vi "Main v1.6.vi"() -> ()   [LabVIEW 2017]
doc: "v0.85:\n- Counts for rejects and total\n\nv0.5:\n\n- Added Reject to Manual Mode\n- Send reject pallet cluster during manual mode\n- Run continuous manual happens only when no error has occured"
uses:
  Controls/Main Tabs v0.1.ctl
  Controls/Auto.ctl
  RT/Controls/Auto Delays.ctl
  RT/Controls/Auto Times.ctl
  support/Controls/General Para.ctl
  support/Message Queue/Message Cluster.ctl
  Controls/UI Data.ctl
  support/Controls/Auto Stats.ctl
  Controls/Logging FGV.ctl
  support/Message Queue/Enqueue Message (Single).vi
  GV/Maintenance GV.vi
  <vilib>/Utility/error.llb/Error Cluster From Error Code.vi
  <vilib>/ErrorRing/Error Ring.xnode
  support/Message Queue/Message Queue.lvlib
  support/User Event - Stop/User Event - Stop.lvlib
panel:
  in  "dup Message Queue":refnum<queue>
  out "path":path
  in  "General Para 2":T1={"Max. Cons."=5.0, "Offset 1"=0.0, "Offset 2"=0.0, "Offset 3"=0.0, "Offset 4"=-0.6, "OutputPause"=500.0, "RejectPause"=500.0} caption="General Para" {"Offset 4" format="%.2f"; "Offset 3" format="%.2f"; "Offset 2" format="%.2f"; "Offset 1" format="%.2f"}
  in  "Auto Para 2":T2={"Agitator Delays"=[250, 600], "TF Delays"=[400, 800, 2, 8000], "Insertion Delays"=[100, 400], "Cutting Delays"=[200, 300, 50], "PF Delays"=[300, 8000], "Measur. Delays"=[200.0, 188.9, 1.0], "Reject Delays"=[500], "BF Delays"=[1000, 1000]}
  out "Shutdown?":bool
  out "Boolean 8":bool
  out "Boolean 7":bool
  out "Boolean 6":bool
  out "Boolean 5":bool
  out "Boolean 4":bool
  out "Boolean 3":bool
  out "Boolean 2":bool
  out "Boolean":bool
  in  "Reject Pallets":T3
  out "Date-Time":string caption="Dip-Tube Assembly Automation (HMI) v1.6"
  out "Main Tab":T4
  in  "All IOs":bool
  in  "Autocycle":T5
  in  "Manual":bool
  in  "Parameters":bool
  in  "Maintenance":bool
  in  "General Para":T1={"Max. Cons."=5.0, "Offset 1"=0.0, "Offset 2"=0.0, "Offset 3"=0.0, "Offset 4"=0.0, "OutputPause"=0.0, "RejectPause"=0.0} {"Offset 4" format="%.2f"; "Offset 3" format="%.2f"; "Offset 2" format="%.2f"; "Offset 1" format="%.2f"}
  in  "BF Para":cluster{"Delay 1":u32, "Delay 2":u32}={"Delay 1"=1000, "Delay 2"=1000}
  in  "Reject Para":cluster{"Delay":u32}={"Delay"=400}
  in  "Meas. Para":T6={"Delay"=500.0, "Mean Length"=188.9, "Tolerance"=1.0}
  in  "PF Para":cluster{"Delay":u32, "Timeout":u32}={"Delay"=1000, "Timeout"=1000}
  in  "Tube Feeder Para":T7={"Delay"=400, "Delay 2"=250, "Max Attempts"=250, "Timeout"=8000}
  in  "Cutting Para":T8={"Delay"=400, "Delay 2"=250, "Delay 3"=250}
  in  "Agitator Para":cluster{"Delay":u32, "Timeout":u32}={"Delay"=400, "Timeout"=250}
  in  "Insertion Para":cluster{"Delay 1":u32, "Delay 2":u32}={"Delay 1"=1000, "Delay 2"=1000}
  in  "Save Para":bool
  in  "Home Para":bool
  out "OEE":dbl format="%#.1f"
  out "QUA":dbl=100.0 min=0.0 max=100.0 step=0.1
  in  "Ideal Time":dbl=2.0 min=0.0 max=100.0 step=0.1
  in  "AVL":dbl=100.0 min=0.0 max=100.0 step=0.1
  out "Rejects 2":u32 caption="Rejects"
  in  "Reset MCount":bool
  in  "Enable BF?":bool
  in  "Enable Agitate?":bool
  in  "Enable Reject?":bool
  in  "Toggle Motor":bool
  in  "Continuous?":bool
  in  "Enable Measure?":bool
  in  "Enable Index?":bool
  in  "Enable PF?":bool
  in  "Manual Para":T2={"Agitator Delays"=[400, 250], "TF Delays"=[700, 800, 2], "Insertion Delays"=[100, 500], "Cutting Delays"=[300, 300, 100], "PF Delays"=[250, 30000], "Measur. Delays"=[500.0, 188.9, 1.0], "Reject Delays"=[500], "BF Delays"=[1000, 1000]}
  in  "Enable Cutting?":bool
  in  "Enable Insertion?":bool
  in  "Run Manual":bool
  in  "Enable TF?":bool
  in  "Home Manual":bool
  out "Status 2":T10
  out "Measurements":T11 {"Height 1" format="%#.2f"; "Height 2" format="%#.2f"; "Height 3" format="%#.2f"; "Height 4" format="%#.2f"}
  out "Output Count":u32 caption="Output\nCount"
  out "PRF":dbl=100.0 min=0.0 max=100.0 step=0.1
  in  "ResetRejectCount":bool
  in  "ResetGoodCount":bool
  out "RejectPause":u32 caption="Reject Parts"
  out "GoodPause":u32 caption="Good Parts"
  in  "End Cycle":bool
  out "Statuses":string[][](table)
  in  "All IO":bool
  in  "Stats":bool
  in  "Home AC":bool
  out "Status":string
  out "Good":u32 format="%06.0f"
  out "Cycle Time":dbl format="%0.2f"
  out "Rejects":u32 format="%05.0f"
  in  "View Log":bool
  out "Total Count 2":u32 caption="Total Count"
  out "Avg. Time":dbl caption="Avg. Cycle Time (s)" format="%#.3f"
  out "Output Chart":cluster{"Good Parts":u32, "Reject Parts":u32}(graph)
  out "Reject Count":u32
  out "Good Count":u32
  out "Total Time":dbl caption="Effective Cycle Time (s)" format="%#.3f"
  out "Time Chart":T12(graph)
  out "OEE Chart":T13(graph)
  out "Timestamp":string caption="Date & Timestamp"
  out "Latest Measure.":T14 caption="Latest Measurements" {"Length 1 (mm)" format="%#.2f"}
  out "Auto Times":T9
  in  "Back Stats":bool
  out "OEE 2":T13 caption="Latest Measurements" {"AVL" format="%#.1f"; "PRF" format="%#.1f"; "QUA" format="%#.1f"; "OEE" format="%#.1f"}
  out "Measurement Chart":T15(graph)
  in  "Home IOs":bool
  in  "Back IO":bool
  out "IAS 4":dbl format="%#.3f"
  out "IAS 3":dbl format="%#.3f"
  out "IAS 2":dbl format="%#.3f"
  out "IAS 1":dbl format="%#.3f"
  out "DI 1":T16
  out "DI 2":T17
  out "DO 1":T18
  in  "Exit":bool
  in  "Shutdown":bool
  # "HARMONY VISION DIP-TUBE ASSEMBLY AUTOMATION"
  # "Auto-Pause after"
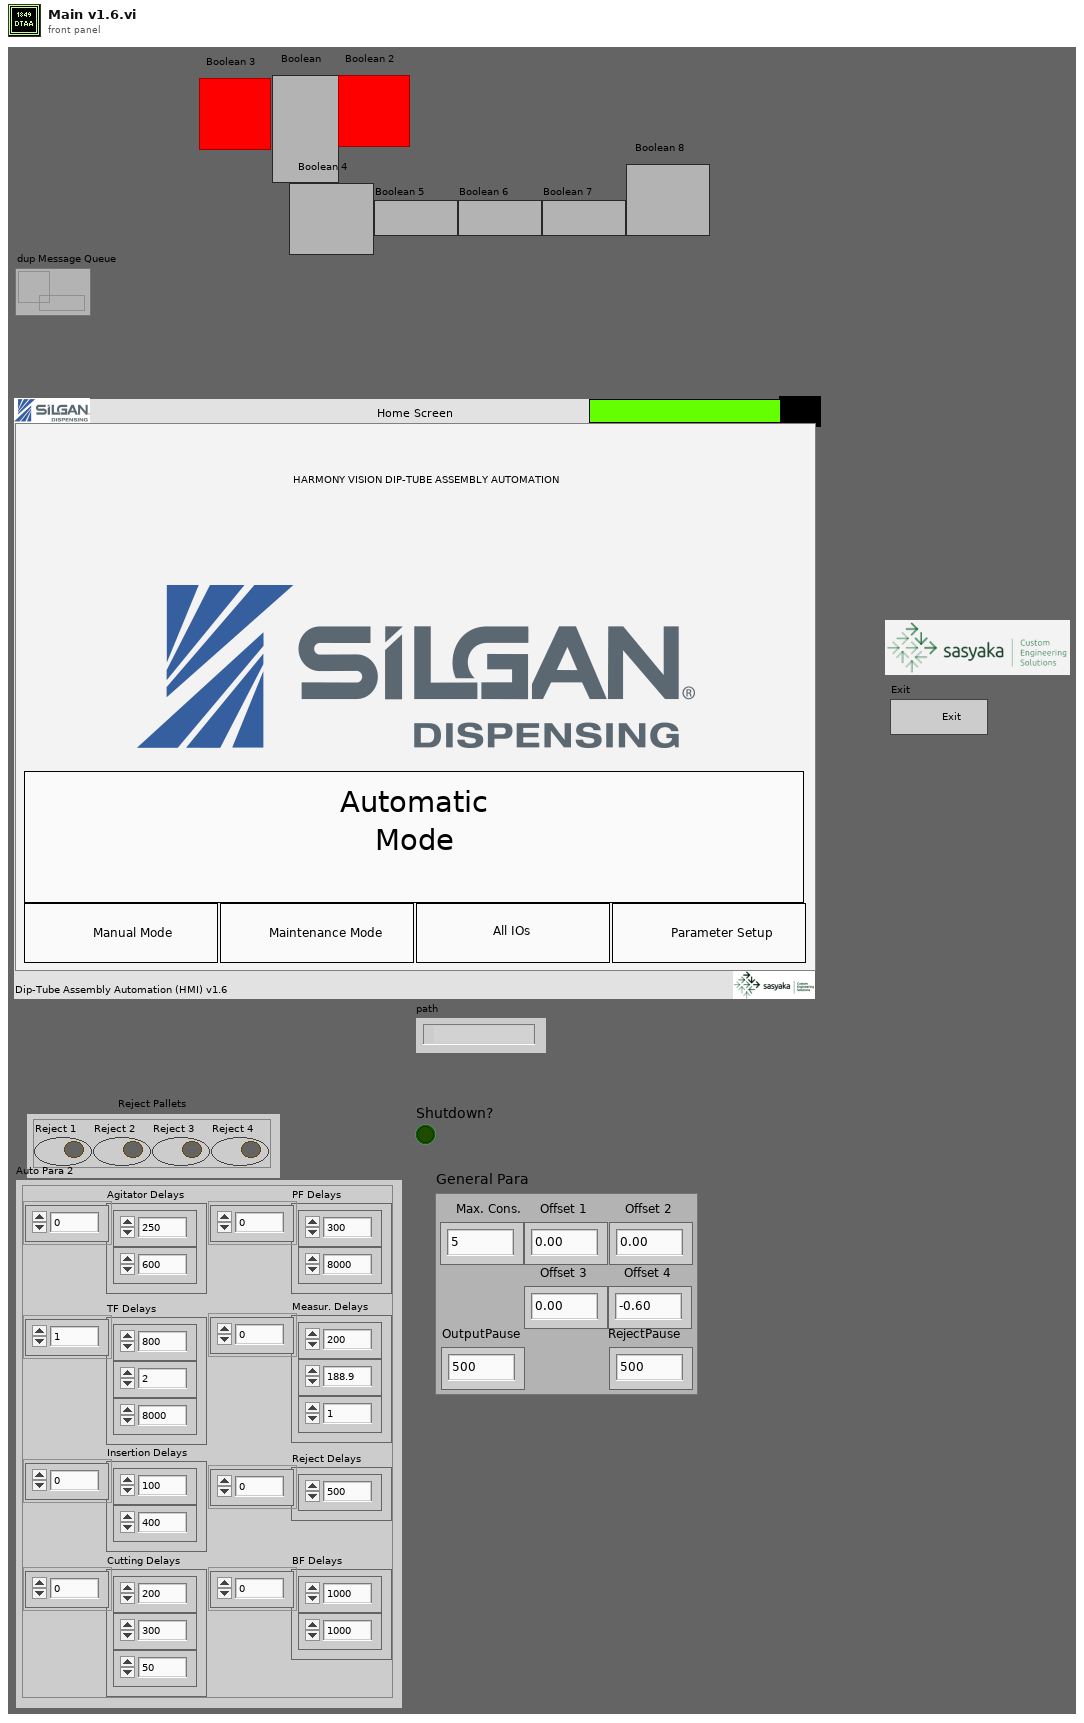
[diagram p1: front panel]
types:
  T1 = typedef "General Para.ctl" = cluster{"Max. Cons.":dbl, "Offset 1":dbl, "Offset 2":dbl, "Offset 3":dbl, "Offset 4":dbl, "OutputPause":dbl, "RejectPause":dbl}
  T2 = typedef "Auto Delays.ctl" = cluster{"Agitator Delays":u32[], "TF Delays":u32[], "Insertion Delays":u32[], "Cutting Delays":u32[], "PF Delays":u32[], "Measur. Delays":dbl[], "Reject Delays":u32[], "BF Delays":u32[]}
  T3 = cluster{"Reject 1":bool, "Reject 2":bool, "Reject 3":bool, "Reject 4":bool}
  T4 = typedef "Main Tabs v0.1.ctl" = enum32{"Home Screen", "Parameter Setup", "Manual Mode", "Autocycle", "Autocycle Statistics", "Autocycle IOs"}
  T5 = typedef "Auto.ctl" = bool
  T6 = cluster{"Delay":dbl, "Mean Length":dbl, "Tolerance":dbl}
  T7 = cluster{"Delay":u32, "Delay 2":u32, "Max Attempts":u32, "Timeout":u32}
  T8 = cluster{"Delay":u32, "Delay 2":u32, "Delay 3":u32}
  T9 = typedef "Auto Times.ctl" = cluster{"Index Time":u32, "TF Time":u32, "Insertion Time":u32, "Cutting Time":u32, "PF Time":u32, "Meas. Time":u32, "Reject Time":u32}
  T10 = cluster{"Auto Times":T9, "error out":errorcluster}
  T11 = cluster{"Height 1":dbl, "Height 2":dbl, "Height 3":dbl, "Height 4":dbl}
  T12 = cluster{"Index":dbl, "TF":dbl, "Insert":dbl, "Cutting":dbl, "PF":dbl, "Measure.":dbl, "Reject":dbl, "Avg. Cycle Time":dbl}
  T13 = cluster{"AVL":dbl, "PRF":dbl, "QUA":dbl, "OEE":dbl}
  T14 = cluster{"Length 1 (mm)":dbl, "Pallet 2 (mm)":dbl, "Pallet 3 (mm)":dbl, "Pallet 4 (mm)":dbl}
  T15 = cluster{"1":dbl, "2":dbl, "3":dbl, "4":dbl, "4":dbl, "4":dbl}
  T16 = cluster{"Machine_ON":bool, "E_stop ":bool, "SW_Pressure":bool, "SW_Start ":bool, "SW_Reset":bool, "SW_Stop":bool, "SW_Door":bool, "RS_Index_Rotary_CW":bool, "RS_Index_Rotary_CCW":bool, "RS_Index_Stopper _Rear":bool, "RS_Index_Output_Separator_Rear":bool, "PES_Index_Pallet_Sensor":bool, "PES_Index_Output_Part Sensor":bool, "ICS_BF_Low_Level_1":bool, "ICS_BF_Low_Level_2":bool, "ICS_BF_Pump_CNVR_Full_1":bool, "ICS_BF_Pump_CNVR_Full_2":bool, "ICS_BF_Pump_CNVR_Full_3":bool, "ICS_BF_Pump_CNVR_Full_4":bool, "PES_PC_Pump Presence_1":bool, "PES_PC_Pump Presence_2":bool, "PES_PC_Pump Presence_3":bool, "PES_PC_Pump Presence_4":bool, "RS_PC_Gating_Front":bool, "PES_Pump_Interference":bool, "PES_TF_Low_Level":bool, "PES_Tube Presence_1":bool, "PES_Tube Presence_2":bool, "PES_Tube Presence_3":bool, "PES_Tube Presence_4":bool, "DI1.30":bool, "DI1.31":bool}
  T17 = cluster{"RS_Agitatator_1_Rear ":bool, "RS_Agitatator_2_Rear ":bool, "RS_TF_Gating CYL_Rear":bool, "RS_Insertion_1_Rear":bool, "RS_Insertion_1_Front":bool, "RS_Insertion _2_Rear":bool, "RS_Insertion _2_Front":bool, "RS_Insertion _3_Rear":bool, "RS_Insertion _3_Front":bool, "RS_Insertion _4_Rear":bool, "RS_Insertion _4_Front":bool, "RS_Insertion_Clamp_Rear":bool, "RS_Cutting_Rear":bool, "RS_Cutting_Clamp _Rear":bool, "RS_Measurement_1_Rear":bool, "RS_Measurement_2_Rear":bool, "RS_Measurement_3_Rear":bool, "RS_Measurement_4_Rear":bool, "DI2.18":bool, "RS_Rejection_1_Rear":bool, "RS_Rejection_2_Rear":bool, "RS_Rejection_3_Rear":bool, "RS_Rejection_4_Rear":bool, "DI2.23":bool, "DI2.24":bool, "DI2.25":bool, "DI2.26":bool, "DI2.27":bool, "DI2.28":bool, "DI2.29":bool, "DI2.30":bool, "DI2.31":bool}
  T18 = cluster{"TL_Red":bool, "TL_Orange":bool, "TL_Green":bool, "TL_Buzzer":bool, "SOL_Index_Rotary_CW":bool, "SOL_Index_Rotary_CCW":bool, "SOL_Index_Stopper_Rear":bool, "SOL_OutputSeparator_Rear":bool, "Bowl  Feeder_ ON 1":bool, "Pump_CNVR_Motor _ON":bool, "SOL_PC_Gating_CYL_Rear":bool, "SOL_Tube_Feed_Agitatator":bool, "SOL_Tube_Feed_Gating_CYL":bool, "SOL_Insertion _CYL":bool, "SOL_Insertion_Clamp_CYL":bool, "SOL_Cutting_CYL":bool, "SOL_Cutting_Clamp_CYL":bool, "SOL_Insertion_Air_Nozzle":bool, "SOL_Measurement_CYL":bool, "DO1.19":bool, "SOL_Rejection CYL_1":bool, "SOL_Rejection CYL_2":bool, "SOL_Rejection CYL_3":bool, "SOL_Rejection CYL_4":bool, "Bowl  Feeder_ ON 2":bool, "SOL_BF_BlowerON":bool, "SOL_BF1_Track1":bool, "SOL_BF1_Track2":bool, "SOL_BF2_Track1":bool, "SOL_BF2_Track2":bool, "DO1.30":bool, "DO1.31":bool}
  T19 = typedef "UI Data.ctl" = cluster{"Main Tab":refnum<vi>}
  T20 = typedef "Message Queue.lvlib/All Message Queues.ctl" = cluster{"UI":refnum<queue>}
  T21 = enum8{"Enabled", "Disabled", "Disabled and Grayed Out"}
  T22 = cluster{"Array":string[][], "Machine Status":string}
  T23 = typedef "Logging FGV.ctl" = enum16{"Start Shift", "Log Index", "Read Shift", "Close Shift"}
  T24 = typedef "Auto Stats.ctl" = cluster{"Time-Stamp":timestamp, "Auto Times":T9, "Measurements":cluster{"1":dbl, "2":dbl, "3":dbl, "4":dbl}, "Outputs":cluster{"Good Parts":u32, "Reject Parts":u32}, "Cycle Time":dbl, "Remarks":string}
  T25 = cluster{"Auto Times":T9, "Results":cluster{"Measurements":cluster{"1":dbl, "2":dbl, "3":dbl, "4":dbl}, "Reject Pallets":cluster{"Reject 1":bool, "Reject 2":bool, "Reject 3":bool, "Reject 4":bool}}, "OutputCount":u32, "error out":errorcluster}
  T26 = enum8{"Information", "Error", "Successful", "Tips"}
  T27 = cluster{"Agitator Delays[0]":u32, "Agitator Delays[1]":u32}
  T28 = cluster{"TF Delays[0]":u32, "TF Delays[1]":u32, "TF Delays[2]":u32, "TF Delays[3]":u32}
  T29 = cluster{"Insertion Delays[0]":u32, "Insertion Delays[1]":u32}
  T30 = cluster{"Cutting Delays[0]":u32, "Cutting Delays[1]":u32, "Cutting Delays[2]":u32}
  T31 = cluster{"Measur. Delays[0]":dbl, "Measur. Delays[1]":dbl, "Measur. Delays[2]":dbl}
  T32 = typedef "All Inputs.ctl" = cluster{"DI 1":cluster{"Machine_ON":bool, "E_stop ":bool, "SW_Pressure":bool, "SW_Start ":bool, "SW_Reset":bool, "SW_Stop":bool, "SW_Door":bool, "RS_Index_Rotary_CW":bool, "RS_Index_Rotary_CCW":bool, "RS_Index_Stopper _Rear":bool, "RS_Cutting_DNClamp _Rear":bool, "PES_Index_Pallet_Sensor":bool, "PES_Index_Output_Part Sensor":bool, "ICS_BF_Low_Level_1":bool, "ICS_BF_Low_Level_2":bool, "ICS_BF_Pump_CNVR_Full_1":bool, "ICS_BF_Pump_CNVR_Full_2":bool, "ICS_BF_Pump_CNVR_Full_3":bool, "ICS_BF_Pump_CNVR_Full_4":bool, "PES_PC_Pump Presence_1":bool, "PES_PC_Pump Presence_2":bool, "PES_PC_Pump Presence_3":bool, "PES_PC_Pump Presence_4":bool, "RS_PC_Gating_Front":bool, "PES_Pump_Interference":bool, "PES_TF_Low_Level":bool, "PES_Tube Presence_1":bool, "PES_Tube Presence_2":bool, "PES_Tube Presence_3":bool, "PES_Tube Presence_4":bool, "DI1.30":bool, "DI1.31":bool}, "DI 2":cluster{"RS_Agitatator_1_Rear ":bool, "RS_Agitatator_2_Rear ":bool, "RS_TF_Gating CYL_Rear":bool, "RS_Insertion_1_Rear":bool, "RS_Insertion_1_Front":bool, "RS_Insertion _2_Rear":bool, "RS_Insertion _2_Front":bool, "RS_Insertion _3_Rear":bool, "RS_Insertion _3_Front":bool, "RS_Insertion _4_Rear":bool, "RS_Insertion _4_Front":bool, "RS_Insertion_Clamp_Rear":bool, "RS_Cutting_Rear":bool, "RS_Cutting_UPClamp _Rear":bool, "RS_Measurement_1_Rear":bool, "RS_Measurement_2_Rear":bool, "RS_Measurement_3_Rear":bool, "RS_Measurement_4_Rear":bool, "RS_Measure_Clamp_Rear":bool, "RS_Rejection_1_Rear":bool, "RS_Rejection_2_Rear":bool, "RS_Rejection_3_Rear":bool, "RS_Rejection_4_Rear":bool, "DI2.23":bool, "DI2.24":bool, "DI2.25":bool, "DI2.26":bool, "DI2.27":bool, "DI2.28":bool, "DI2.29":bool, "DI2.30":bool, "DI2.31":bool}, "IAS 1":dbl, "IAS 2":dbl, "IAS 3":dbl, "IAS 4":dbl, "DO 1":cluster{"TL_Red":bool, "TL_Orange":bool, "TL_Green":bool, "TL_Buzzer":bool, "SOL_Index_Rotary_CW":bool, "SOL_Index_CNVR_Rotary_CCW":bool, "SOL_Index_CNVR_Stopper_Rear":bool, "SOL_Index_CNVR_Output _Separator _Rear":bool, "Bowl  Feeder_ ON 1":bool, "Pump_CNVR_Motor _ON":bool, "SOL_PC_Gating_CYL_Rear":bool, "SOL_Tube_Feed_Agitatator":bool, "SOL_Tube_Feed_Gating_CYL":bool, "SOL_Insertion _CYL":bool, "SOL_Insertion_Clamp_CYL":bool, "SOL_Cutting_CYL":bool, "SOL_Cutting_Clamp_CYL":bool, "SOL_Insertion_Air_Nozzle":bool, "SOL_Measurement_CYL":bool, "DO1.19":bool, "SOL_Rejection CYL_1":bool, "SOL_Rejection CYL_2":bool, "SOL_Rejection CYL_3":bool, "SOL_Rejection CYL_4":bool, "Bowl  Feeder_ ON 2":bool, "SOL_BF_BlowerON":bool, "SOL_BF1_Track1":bool, "SOL_BF1_Track2":bool, "SOL_BF2_Track1":bool, "SOL_BF2_Track2":bool, "DO1.30":bool, "DO1.31":bool}}
  T33 = cluster{"Machine_ON":bool, "E_stop ":bool, "SW_Pressure":bool, "SW_Start ":bool, "SW_Reset":bool, "SW_Stop":bool, "SW_Door":bool, "RS_Index_Rotary_CW":bool, "RS_Index_Rotary_CCW":bool, "RS_Index_Stopper _Rear":bool, "RS_Cutting_DNClamp _Rear":bool, "PES_Index_Pallet_Sensor":bool, "PES_Index_Output_Part Sensor":bool, "ICS_BF_Low_Level_1":bool, "ICS_BF_Low_Level_2":bool, "ICS_BF_Pump_CNVR_Full_1":bool, "ICS_BF_Pump_CNVR_Full_2":bool, "ICS_BF_Pump_CNVR_Full_3":bool, "ICS_BF_Pump_CNVR_Full_4":bool, "PES_PC_Pump Presence_1":bool, "PES_PC_Pump Presence_2":bool, "PES_PC_Pump Presence_3":bool, "PES_PC_Pump Presence_4":bool, "RS_PC_Gating_Front":bool, "PES_Pump_Interference":bool, "PES_TF_Low_Level":bool, "PES_Tube Presence_1":bool, "PES_Tube Presence_2":bool, "PES_Tube Presence_3":bool, "PES_Tube Presence_4":bool, "DI1.30":bool, "DI1.31":bool}
  T34 = cluster{"RS_Agitatator_1_Rear ":bool, "RS_Agitatator_2_Rear ":bool, "RS_TF_Gating CYL_Rear":bool, "RS_Insertion_1_Rear":bool, "RS_Insertion_1_Front":bool, "RS_Insertion _2_Rear":bool, "RS_Insertion _2_Front":bool, "RS_Insertion _3_Rear":bool, "RS_Insertion _3_Front":bool, "RS_Insertion _4_Rear":bool, "RS_Insertion _4_Front":bool, "RS_Insertion_Clamp_Rear":bool, "RS_Cutting_Rear":bool, "RS_Cutting_UPClamp _Rear":bool, "RS_Measurement_1_Rear":bool, "RS_Measurement_2_Rear":bool, "RS_Measurement_3_Rear":bool, "RS_Measurement_4_Rear":bool, "RS_Measure_Clamp_Rear":bool, "RS_Rejection_1_Rear":bool, "RS_Rejection_2_Rear":bool, "RS_Rejection_3_Rear":bool, "RS_Rejection_4_Rear":bool, "DI2.23":bool, "DI2.24":bool, "DI2.25":bool, "DI2.26":bool, "DI2.27":bool, "DI2.28":bool, "DI2.29":bool, "DI2.30":bool, "DI2.31":bool}
  T35 = cluster{"TL_Red":bool, "TL_Orange":bool, "TL_Green":bool, "TL_Buzzer":bool, "SOL_Index_Rotary_CW":bool, "SOL_Index_CNVR_Rotary_CCW":bool, "SOL_Index_CNVR_Stopper_Rear":bool, "SOL_Index_CNVR_Output _Separator _Rear":bool, "Bowl  Feeder_ ON 1":bool, "Pump_CNVR_Motor _ON":bool, "SOL_PC_Gating_CYL_Rear":bool, "SOL_Tube_Feed_Agitatator":bool, "SOL_Tube_Feed_Gating_CYL":bool, "SOL_Insertion _CYL":bool, "SOL_Insertion_Clamp_CYL":bool, "SOL_Cutting_CYL":bool, "SOL_Cutting_Clamp_CYL":bool, "SOL_Insertion_Air_Nozzle":bool, "SOL_Measurement_CYL":bool, "DO1.19":bool, "SOL_Rejection CYL_1":bool, "SOL_Rejection CYL_2":bool, "SOL_Rejection CYL_3":bool, "SOL_Rejection CYL_4":bool, "Bowl  Feeder_ ON 2":bool, "SOL_BF_BlowerON":bool, "SOL_BF1_Track1":bool, "SOL_BF1_Track2":bool, "SOL_BF2_Track1":bool, "SOL_BF2_Track2":bool, "DO1.30":bool, "DO1.31":bool}
  T36 = cluster{"Index":dbl, "TF":dbl, "Insert":dbl, "Cutting":dbl, "PF":dbl, "Measure.":dbl, "Reject":dbl}
  T37 = cluster{"1":dbl, "2":dbl, "3":dbl, "4":dbl, dbl, dbl}
  T38 = cluster{"Manual Para":T2, "Reject Pallets":cluster{"Reject 1":bool, "Reject 2":bool, "Reject 3":bool, "Reject 4":bool}}
  T39 = cluster{"Measurements":cluster{"1":dbl, "2":dbl, "3":dbl, "4":dbl}, "Reject Pallets":cluster{"Reject 1":bool, "Reject 2":bool, "Reject 3":bool, "Reject 4":bool}}
  T40 = cluster{"Reject Pallets":cluster{"Reject 1":bool, "Reject 2":bool, "Reject 3":bool, "Reject 4":bool}, "Measurements":cluster{"1":dbl, "2":dbl, "3":dbl, "4":dbl}}
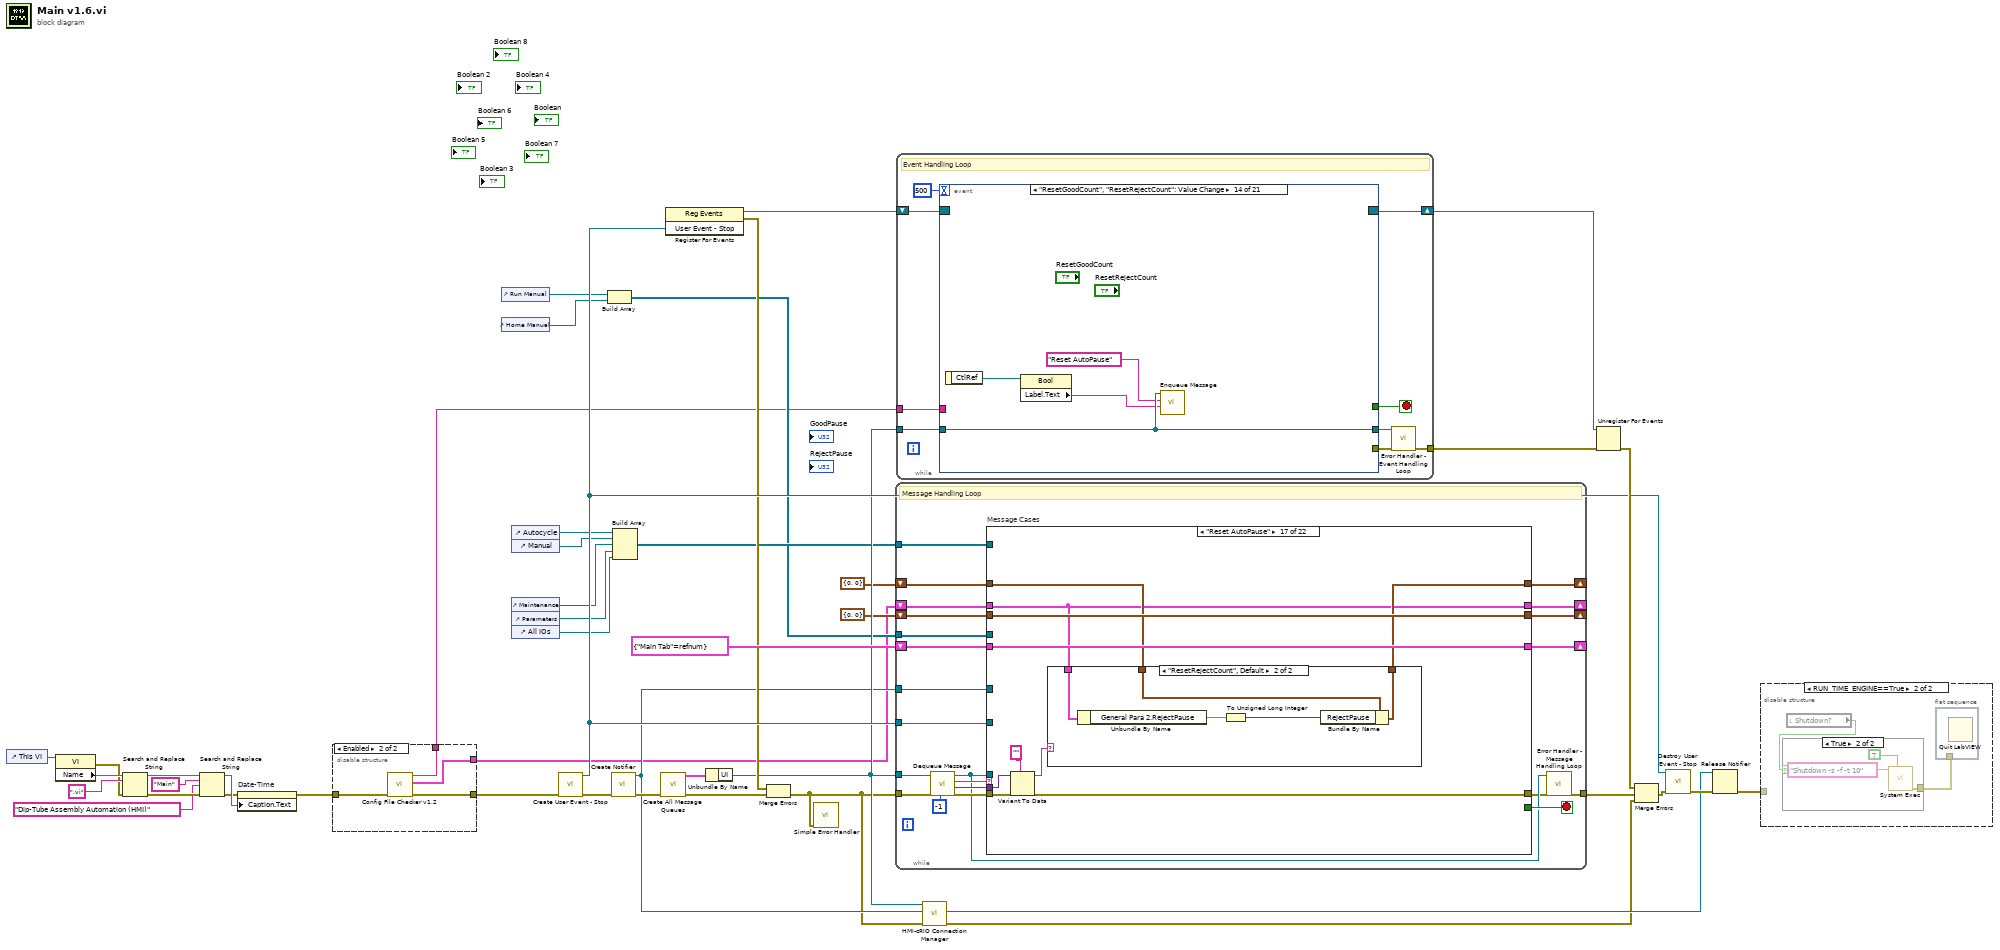
[diagram p0: block diagram]
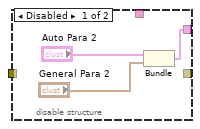
[diagram p2: hidden frame]
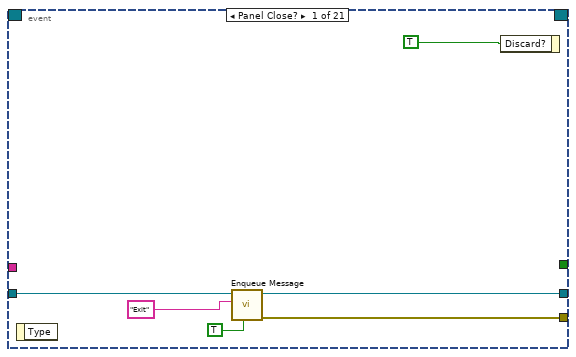
[diagram p3: hidden frame]
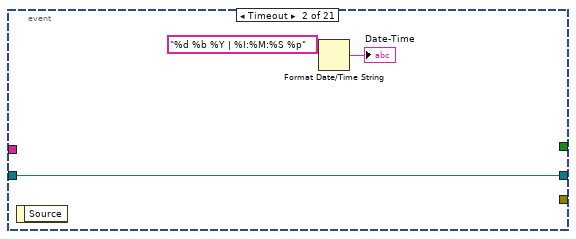
[diagram p4: hidden frame]
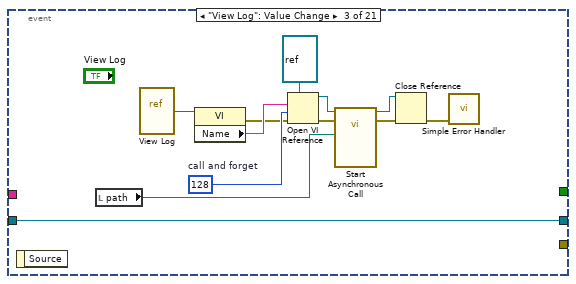
[diagram p5: hidden frame]
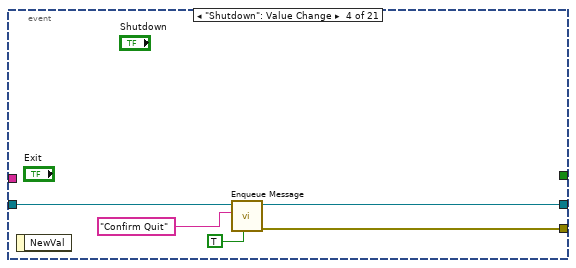
[diagram p6: hidden frame]
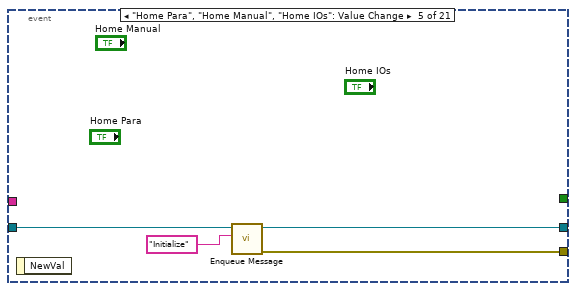
[diagram p7: hidden frame]
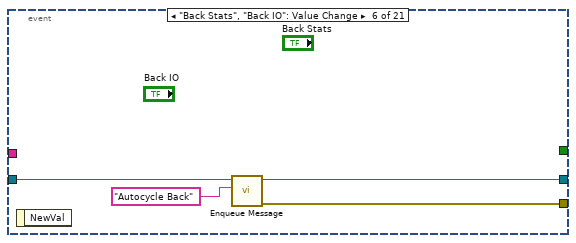
[diagram p8: hidden frame]
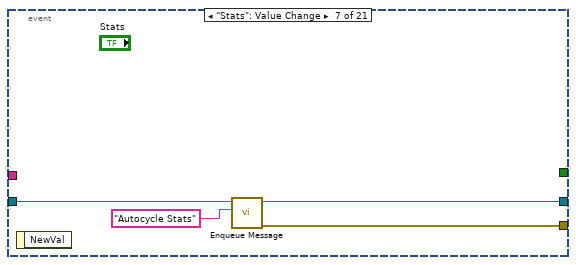
[diagram p9: hidden frame]
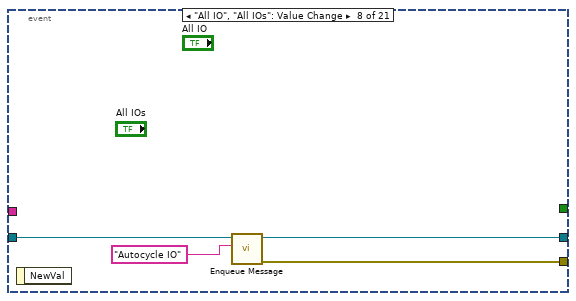
[diagram p10: hidden frame]
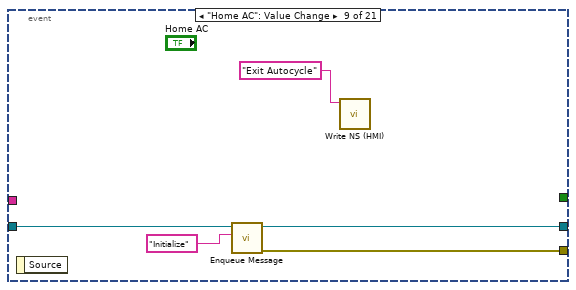
[diagram p11: hidden frame]
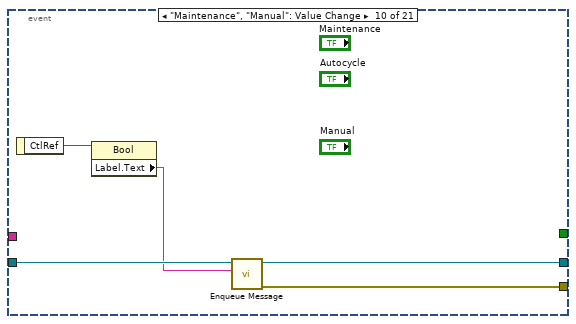
[diagram p12: hidden frame]
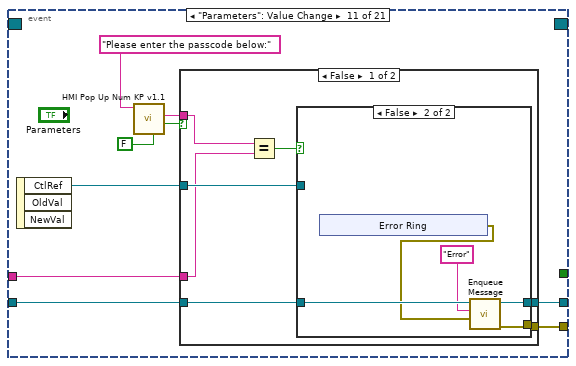
[diagram p13: hidden frame]
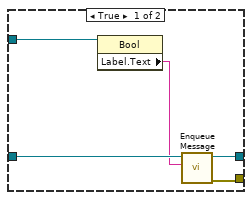
[diagram p14: hidden frame]
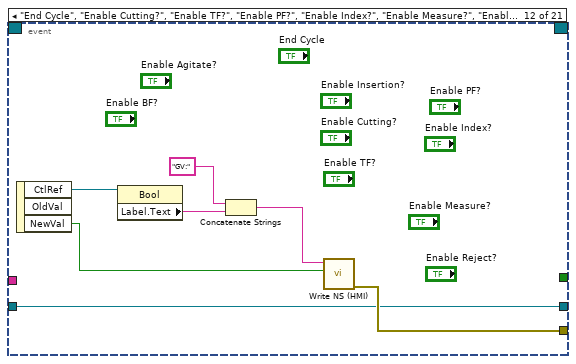
[diagram p16: hidden frame]
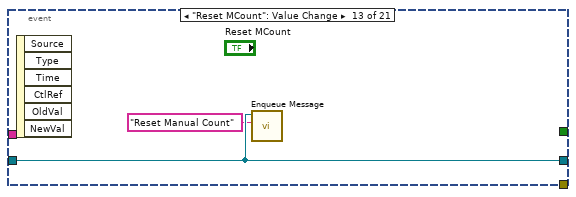
[diagram p17: hidden frame]
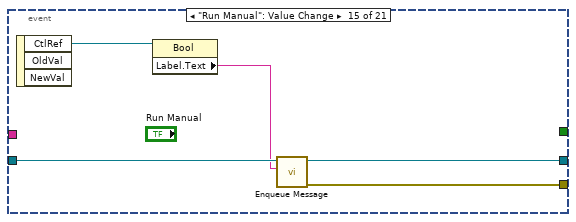
[diagram p18: hidden frame]
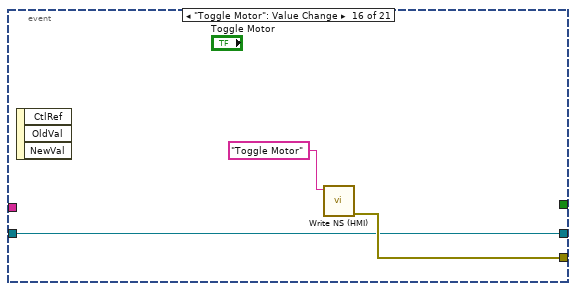
[diagram p19: hidden frame]
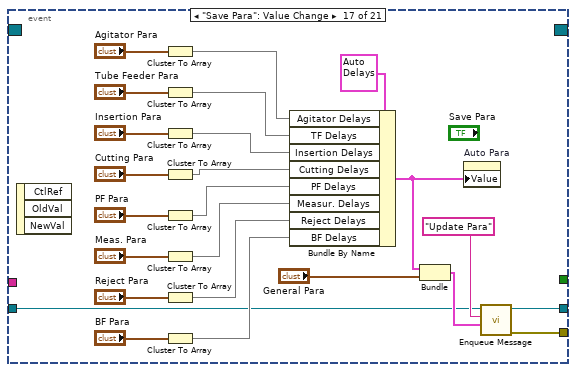
[diagram p20: hidden frame]
diagram:
  n1 = control-ref of="This VI"() -> (w16:refnum<vi>)
  n2 = property class="VI"(reference=w16) -> (error out=w15:errorcluster, "Name"=w22:string)  [unwired: 1 in, 1 out]
  n3 = Search and Replace String(input string=w22, search string=".vi", error in=w15) -> (result string=w20:string, error out=w19:errorcluster)  [unwired: 5 in, 2 out]
  n4 = Search and Replace String(input string=w20, search string="Main", replace string="Dip-Tube Assembly Automation (HMI)" ("replace string (\"\")"), error in=w19) -> (result string=w14:string, error out=w13:errorcluster)  [unwired: 4 in, 2 out]
  n5 = property on="Date-Time" class="Str"(error in=w13, "Caption.Text"=w14) -> (error out=w6:errorcluster)  [unwired: 1 in, 1 out]
  n6 = disable-structure shown="Enabled" {
    disable-tunnel: [w46 w52] -> w4
    disable-tunnel: w6 -> [_ w51]
    disable-tunnel: [_ w50] -> w5
    disable-tunnel: [_ w49] -> w3
    frame Disabled {
      n7 = Bundle("Auto Para 2"="Auto Para 2", "General Para 2"="General Para 2") -> (w46:cluster{"Auto Para 2":T2, "General Para 2":T1})  [unwired: 1 in]
    }
    frame Enabled {
      n8 = call "Config File Checker v1.2.vi"("Error In"=w51) -> ("error out"=w50:errorcluster, "All Para"=w52:cluster{"Auto Para":T2, "General Para 2":T1}, "password"=w49:string)  [unwired: 7 in, 1 out]
    }
  }
  n9 = control-ref of="Run Manual"() -> (w12:refnum<vi>)
  n10 = control-ref of="Home Manual"() -> (w11:refnum<vi>)
  n11 = control-ref of="Autocycle"() -> (w27:refnum<vi>)
  n12 = control-ref of="Manual"() -> (w26:refnum<vi>)
  n13 = control-ref of="Maintenance"() -> (w25:refnum<vi>)
  n14 = control-ref of="Parameters"() -> (w24:refnum<vi>)
  n15 = control-ref of="All IOs"() -> (w7:refnum<vi>)
  n16 = call "Create User Event - Stop.vi"("error in (no error)"=w5) -> ("error out"=w33:errorcluster, "User Event - Stop"=w36:refnum<user-event>)  [unwired: 9 in]
  n17 = Build Array(w12, w11) -> (w10:refnum<vi>[])
  n18 = call "Create Notifier.vi"("error in (no error)"=w33) -> ("error out"=w32:errorcluster, "notifier out"=w8:refnum<notifier>)  [unwired: 9 in]
  n19 = Build Array(w27, w26, w25, w24, w7) -> (w23:refnum<vi>[])
  n20 = call "Create All Message Queues.vi"("error in (no error)"=w32) -> ("error out"=w45:errorcluster, "Message Queues out"=w44:T20)  [unwired: 9 in]
  n21 = register-events(w36) -> (reference out=w37:refnum<event-registration>, error out=w35:errorcluster)  [unwired: 2 in]
  n22 = Unbundle By Name(w44) -> ("UI"=w34:refnum<queue>)
  n23 = Merge Errors(w35, w45) -> (w2:errorcluster)
  n24 = call <vilib>:"Simple Error Handler.vi"("error in (no error)"=w2) -> ()  [unwired: 4 in, 5 out]
  n25 = while {
    tunnel: w34 -> [w67]
    shift-right: [w74] -> _
    shift-left: T19 {"Main Tab"=refnum} ("Data Cluster") -> [w57]
    tunnel: w36 -> [w72]
    tunnel: w2 -> [w71]
    tunnel: [w65] -> w43
    tunnel: w8 -> [w62]
    tunnel: w23 -> [w61]
    tunnel: w10 -> [w60]
    shift-right: [w58] -> _
    shift-left: cluster{"OutputCount":u32, "RejectCount":u32} {"OutputCount"=0, "RejectCount"=0} -> [w59]
    shift-right: [w55] -> _
    shift-left: w4 -> [w56]
    shift-right: [w53] -> _
    shift-left: cluster{"GoodPause":u32, "RejectPause":u32} {"GoodPause"=0, "RejectPause"=0} ("cluster") -> [w54]
    stop <- w73 stop-if-true
    # "Message Handling Loop"
    n26 = call "Dequeue Message.vi"("timeout"=-1, "error in (no error)"=w71, "Message Queue"=w67) -> ("error out"=w70:errorcluster, "Message Data"=w68:variant, "Message"=w69:string, "dup Message Queue"=w66:refnum<queue>)  [unwired: 5 in]
    n27 = case "Message Cases" shown="\"Reset AutoPause\"" w69 {
      selector: w69 -> [_ _ _ _ _ _ _ _ _ _ _ _ _ _ _ _ _ _ _ _ _ w483]
      tunnel: w66 -> [_ _ _ _ _ _ _ _ _ w218 w228 _ w270 _ w352 _ _ _ _ w452 w479 _]
      tunnel: w70 -> [w84 w89 w105 w135 w152 w170 w181 w204 w211 w220 w236 w266 w314 w326 w360 w372 w380 w417 w442 w456 w472 _]
      tunnel: [w84 w88 w94 w135 w147 w170 w180 w204 w211 w219 w235 w267 w315 w328 w351 w372 w379 w412 w437 w454 w475 w484] -> w64
      tunnel: w57 -> [w83 w90 w107 w139 w154 w169 w177 w208 w215 w225 w233 w268 w316 w329 w361 w371 w382 w416 w441 w455 w478 w485]
      tunnel: [w82 w90 w107 w139 w154 w169 w177 w208 w215 w225 w233 w268 w316 w329 w361 w371 w382 w416 w441 w455 w478 w485] -> w74
      tunnel: [_ _ _ _ _ _ _ _ _ _ _ _ _ _ _ _ _ _ _ _ TRUE _] -> w73
      tunnel: w68 -> [_ _ w104 _ w151 _ _ _ _ _ _ w265 w313 _ w359 _ w378 w415 w440 _ w469 _]
      tunnel: w72 -> [_ _ _ _ _ _ _ _ _ _ _ _ _ _ _ _ _ _ _ _ w474 _]
      tunnel: w62 -> [_ _ _ _ _ _ _ _ _ _ _ _ _ _ _ _ _ _ _ _ w468 _]
      tunnel: w61 -> [_ _ w100 _ _ _ _ _ _ _ _ _ _ _ _ _ _ _ _ _ _ _]
      tunnel: w60 -> [_ _ _ _ _ _ _ _ _ _ _ _ _ w323 w357 _ _ _ _ _ _ _]
      tunnel: w59 -> [w79 w87 w96 w136 w153 w158 w182 w205 w212 w222 w237 w263 w311 w319 w350 _ w381 w411 w436 w451 w465 w482]
      tunnel: [w79 w87 w96 w136 w153 w158 w182 w205 w212 w222 w237 w263 w311 w319 w345 cluster{"OutputCount":u32, "RejectCount":u32} {"OutputCount"=0, "RejectCount"=0} w381 w411 w436 w451 w465 w482] -> w58
      tunnel: w56 -> [w76 w86 w93 w116 _ w157 w176 w203 w210 w217 w227 w252 w280 w318 w333 w368 w373 w394 w419 w444 w464 w481]
      tunnel: [w76 w86 w93 w116 w146 w157 w176 w203 w210 w217 w227 w252 w280 w318 w333 w368 w373 w394 w419 w444 w464 w481] -> w55
      tunnel: w54 -> [w75 w85 w91 w115 w140 w155 w173 w202 w209 w216 w226 w251 w272 w317 w332 w367 w375 w393 w418 w443 w463 w480]
      tunnel: [w75 w85 w91 w115 w140 w155 w174 w202 w209 w216 w226 w251 w271 w317 w332 w367 w374 w393 w418 w443 w463 w480] -> w53
      frame "Initialize" {
        # "Initialize - All initialization work should take place in this message, since other loops can potentially enqueue messages that execute immediately after this one."
        n28 = control-ref of="Main Tab"() -> (w81:refnum<vi>)
        n29 = Bundle By Name(cluster=w83, "Main Tab"=w81) -> (w82:T19)
        n30 = property on="Home IOs" class="Bool"("Visible"=TRUE) -> ()  [unwired: 2 in, 2 out]
        n31 = property on="Back IO" class="Bool"("Visible"=FALSE) -> ()  [unwired: 2 in, 2 out]
        "Main Tab" <- Main_Tabs_v0.1."Home Screen" ("Main Tab")
      }
      frame "Maintenance" {
        # "Maintenance"
        n32 = call "Maintenance v0.3.vi"("Error In"=w89) -> ("Error out"=w88:errorcluster)  [unwired: 10 in]
      }
      frame "Connection" {
        n33 = Variant To Data(error in=w105, type=FALSE, Variant=w104) -> (data=w92:bool, error out=w95:errorcluster)
        n34 = Select(t=u32 6618880 ("Text.Text Colors:BG Color"), s=w92, f=u32 16762112 ("Text.Text Colors:BG Color")) -> (s? t:f=w101:u32)
        n35 = property on="Date-Time" class="Str"("Text.BGColor"=w101) -> ()  [unwired: 2 in, 2 out]
        n36 = Select(t=T21."Enabled" ("Disabled"), s=w92, f=T21."Disabled and Grayed Out") -> (s? t:f=w98:T21)
        n37 = for {
          tunnel: w100 -> [w114] mode=indexing
          tunnel: w98 -> [w113]
          n38 = property class="Bool"(reference=w114, "DisabledEnum"=w113) -> ()  [unwired: 1 in, 2 out]
        }
        n39 = case shown="True" w92 {
          tunnel: w95 -> [w108 w111]
          tunnel: [w108 w110] -> w94
          tunnel: w93 -> [_ w109]
          frame False {
          }
          frame True {
            n40 = call "Write NS (HMI).vi"("error in (no error)"=w111, "Message Data"=w109, "Message"="Save Para") -> ("error out"=w110:errorcluster)  [unwired: 8 in]
          }
        }
      }
      frame "Parameters" {
        # "Parameters"
        n41 = Unbundle(w116) -> ("Auto Para"=w118:T2, "General Para 2"=w117:T1)
        n42 = Unbundle By Name(w139) -> ("Main Tab"=w138:refnum<vi>)
        n43 = property on="General Para" class="Clust (strict)"("Value"=w117) -> ()  [unwired: 2 in, 2 out]
        n44 = Unbundle(w118) -> ("Agitator Delays"=w134:u32[], "TF Delays"=w133:u32[], "Insertion Delays"=w132:u32[], "Cutting Delays"=w131:u32[], "PF Delays"=w130:u32[], "Measur. Delays"=w129:dbl[], "Reject Delays"=w128:u32[], "BF Delays"=w127:u32[])
        n45 = property class="TabCtl"(reference=w138, "Value"=Main_Tabs_v0.1."Parameter Setup" ("Main Tab")) -> ()  [unwired: 1 in, 2 out]
        n46 = Array To Cluster(array=w134) -> (cluster=w126:T27)
        n47 = Array To Cluster(array=w133) -> (cluster=w125:T28)
        n48 = Array To Cluster(array=w132) -> (cluster=w124:T29)
        n49 = Array To Cluster(array=w131) -> (cluster=w123:T30)
        n50 = Array To Cluster(array=w130) -> (cluster=w122:cluster{"PF Delays[0]":u32, "PF Delays[1]":u32})
        n51 = Array To Cluster(array=w129) -> (cluster=w121:T31)
        n52 = Array To Cluster(array=w128) -> (cluster=w120:cluster{"Reject Delays[0]":u32})
        n53 = Array To Cluster(array=w127) -> (cluster=w119:cluster{"BF Delays[0]":u32, "BF Delays[1]":u32})
        n54 = property on="Agitator Para" class="Clust (strict)"("Value"=w126) -> ()  [unwired: 2 in, 2 out]
        n55 = property on="Tube Feeder Para" class="Clust (strict)"("Value"=w125) -> ()  [unwired: 2 in, 2 out]
        n56 = property on="Insertion Para" class="Clust (strict)"("Value"=w124) -> ()  [unwired: 2 in, 2 out]
        n57 = property on="Cutting Para" class="Clust (strict)"("Value"=w123) -> ()  [unwired: 2 in, 2 out]
        n58 = property on="PF Para" class="Clust (strict)"("Value"=w122) -> ()  [unwired: 2 in, 2 out]
        n59 = property on="Meas. Para" class="Clust (strict)"("Value"=w121) -> ()  [unwired: 2 in, 2 out]
        n60 = property on="Reject Para" class="Clust (strict)"("Value"=w120) -> ()  [unwired: 2 in, 2 out]
        n61 = property on="BF Para" class="Clust (strict)"("Value"=w119) -> ()  [unwired: 2 in, 2 out]
      }
      frame "Update Para" {
        # "Parameters"
        n62 = Variant To Data(error in=w152, type=cluster{"Auto Para":T2, "General Para":T1} {"Auto Para"={"Agitator Delays"=[], "TF Delays"=[], "Insertion Delays"=[], "Cutting Delays"=[], "PF Delays"=[], "Measur. Delays"=[], "Reject Delays"=[], "BF Delays"=[]}, "General Para"={"Max. Cons."=0.0, "Offset 1"=0.0, "Offset 2"=0.0, "Offset 3"=0.0, "Offset 4"=0.0, "OutputPause"=0.0, "RejectPause"=0.0}} ("cluster"), Variant=w151) -> (data=w146:cluster{"Auto Para":T2, "General Para":T1}, error out=w148:errorcluster)
        n63 = call <vilib>:"Application Directory.vi"() -> ("Application Directory"=w145:path)
        n64 = Build Path(base path=w145, name or relative path="data") -> (appended path=w143:path)
        n65 = Build Path(base path=w143, name or relative path="config.ini") -> (appended path=w142:path)
        n66 = call "Write NS (HMI).vi"("error in (no error)"=w148, "Message Data"=w146, "Message"="Save Para") -> ("error out"=w147:errorcluster)  [unwired: 8 in]
        n67 = call "Write Config v1.1.vi"("All Para"=w146, "file path"=w142) -> ()  [unwired: 8 in, 2 out]
      }
      frame "Manual" {
        # "Parameters"
        n68 = control-ref of="Enable Index?"() -> (w166:refnum<vi>)
        n69 = control-ref of="Enable PF?"() -> (w165:refnum<vi>)
        n70 = control-ref of="Enable Cutting?"() -> (w164:refnum<vi>)
        n71 = control-ref of="Enable Insertion?"() -> (w163:refnum<vi>)
        n72 = control-ref of="Enable TF?"() -> (w162:refnum<vi>)
        n73 = control-ref of="Enable Measure?"() -> (w160:refnum<vi>)
        n74 = Unbundle By Name(w157) -> ("Auto Para"=w156:T2)
        n75 = control-ref of="Enable Reject?"() -> (w159:refnum<vi>)
        n76 = Build Array(w166, w165, w164, w163, w162, w160, w159) -> (w161:refnum<vi>[])
        n77 = property on="Auto Para" class="Clust (strict)"("Value"=w156) -> ()  [unwired: 2 in, 2 out]
        n78 = for {
          tunnel: w161 -> [w172] mode=indexing
          n79 = property class="Bool (strict)"(reference=w172, "Val(Sgnl)"=FALSE ("Value (Signaling)")) -> ()  [unwired: 1 in, 2 out]
        }
        n80 = Unbundle By Name(w169) -> ("Main Tab"=w168:refnum<vi>)
        n81 = property class="TabCtl"(reference=w168, "Value"=Main_Tabs_v0.1."Manual Mode" ("Main Tab")) -> ()  [unwired: 1 in, 2 out]
      }
      frame "Autocycle" {
        # "Parameters"
        n82 = call "Select Model v0.1.vi"() -> ("Cancel out"=w178:bool, "Refresh Indicators?"=w175:bool, "Model out"=w179:string)  [unwired: 9 in]
        n83 = case shown="False" w178 {
          tunnel: w181 -> [w191 w201]
          tunnel: [w198 w201] -> w180
          tunnel: w179 -> [w197 _]
          tunnel: w177 -> [w194 _]
          tunnel: w176 -> [w188 _]
          tunnel: w175 -> [_ _]
          tunnel: [w183 w200] -> w174
          tunnel: w173 -> [_ w200]
          frame False {
            n84 = Unbundle By Name(w194) -> ("Main Tab"=w196:refnum<vi>)
            n85 = Unbundle By Name(w188) -> ("General Para 2.OutputPause"=w187:dbl, "General Para 2.RejectPause"=w186:dbl)
            n86 = call "Write NS (HMI).vi"("error in (no error)"=w191, "Message Data"=w188, "Message"="Save Para") -> ("error out"=w190:errorcluster)  [unwired: 8 in]
            n87 = property class="TabCtl"(reference=w196, "Value"=Main_Tabs_v0.1."Autocycle" ("Main Tab")) -> ()  [unwired: 1 in, 2 out]
            n88 = call "Write NS (HMI).vi"("error in (no error)"=w190, "Message Data"=w197, "Message"="Autocycle") -> ("error out"=w198:errorcluster)  [unwired: 8 in]
            n89 = property on="Home IOs" class="Bool"("Visible"=FALSE) -> ()  [unwired: 2 in, 2 out]
            n90 = property on="Back IO" class="Bool"("Visible"=TRUE) -> ()  [unwired: 2 in, 2 out]
            n91 = To Unsigned Long Integer(number=w186) -> (unsigned 32bit integer=w184:u32)
            n92 = To Unsigned Long Integer(number=w187) -> (unsigned 32bit integer=w185:u32)
            n93 = Bundle(w185, w184) -> (w183:cluster{u32, u32})  [unwired: 1 in]
          }
          frame True {
          }
        }
      }
      frame "Autocycle Back" {
        # "Parameters"
        n94 = Unbundle By Name(w208) -> ("Main Tab"=w207:refnum<vi>)
        n95 = property class="TabCtl"(reference=w207, "Value"=Main_Tabs_v0.1."Autocycle" ("Main Tab")) -> ()  [unwired: 1 in, 2 out]
      }
      frame "Autocycle Stats" {
        # "Parameters"
        n96 = Unbundle By Name(w215) -> ("Main Tab"=w214:refnum<vi>)
        n97 = property class="TabCtl"(reference=w214, "Value"=Main_Tabs_v0.1."Autocycle Statistics" ("Main Tab")) -> ()  [unwired: 1 in, 2 out]
      }
      frame "Autocycle IO" {
        # "Parameters"
        n98 = Unbundle By Name(w225) -> ("Main Tab"=w224:refnum<vi>)
        n99 = property class="TabCtl"(reference=w224, "Value"=Main_Tabs_v0.1."Autocycle IOs" ("Main Tab")) -> ()  [unwired: 1 in, 2 out]
        n100 = call-poly "Enqueue Message.vi"("error in (no error)"=w220, "Message"="Update IO", "Message Queue"=w218) -> ("error out"=w219:errorcluster)  [unwired: 7 in, 1 out]
      }
      frame "Update IO" {
        n101 = Unbundle By Name(w233) -> ("Main Tab"=w234:refnum<vi>)
        n102 = Wait (ms)(milliseconds to wait=u32 200) -> ()  [unwired: 1 out]
        n103 = property class="TabCtl"(reference=w234) -> ("Value"=w232:variant)  [unwired: 1 in, 2 out]
        n104 = Variant To Data(type=Main_Tabs_v0.1."Autocycle IOs" ("Main Tab"), Variant=w232) -> (data=w229:T4)  [unwired: 1 in, 1 out]
        n105 = global read "Maintenance GV.vi" "All IO"() -> (w238:T32)
        n106 = case shown="\"Autocycle IOs\"" w229 {
          tunnel: w236 -> [w246 w249]
          tunnel: [w246 w248] -> w235
          tunnel: w228 -> [_ w247]
          frame Default {
          }
          frame "Autocycle IOs" {
            n107 = call-poly "Enqueue Message.vi"("error in (no error)"=w249, "Message"="Update IO", "Message Queue"=w247) -> ("error out"=w248:errorcluster)  [unwired: 7 in, 1 out]
          }
        }
        n108 = Unbundle(w238) -> ("DI 1"=→"DI 1":T33, "DI 2"=→"DI 2":T34, "IAS 1"=→"IAS 1":dbl, "IAS 2"=→"IAS 2":dbl, "IAS 3"=→"IAS 3":dbl, "IAS 4"=→"IAS 4":dbl, "DO 1"=→"DO 1":T35)
      }
      frame "Update UI" {
        # "Update Display - Convert the message data to a string to display in the Data Display indicator."
        n109 = Variant To Data(error in=w266, type=T22 {"Array"=[], "Machine Status"=""} ("Status Cluster"), Variant=w265) -> (data=w261:T22, error out=w264:errorcluster)
        n110 = Unbundle(w261) -> ("Array"=→"Statuses":string[][], "Machine Status"=w259:string)
        "Status" <- w259
        n111 = Search and Replace String(input string=w259, search string="Autocycle is Running") -> (number of replacements=w257:i32)  [unwired: 6 in, 3 out]
        n112 = Greater Than 0?(x=w257) -> (x > 0?=w255:bool)
        n113 = Select(t=T21."Disabled and Grayed Out" ("Disabled"), s=w255, f=T21."Enabled" ("Disabled")) -> (s? t:f=w254:T21)
        n114 = property on="Home AC" class="Bool"("DisabledEnum"=w254) -> ()  [unwired: 2 in, 2 out]
        n115 = Merge Errors(w264) -> (w267:errorcluster)
      }
      frame "Autocycle Log" {
        # "Update Display - Convert the message data to a string to display in the Data Display indicator."
        n116 = Variant To Data(error in=w314, type=T24 {"Time-Stamp"=timestamp(0 s since 1904-01-01), "Auto Times"={"Index Time"=0, "TF Time"=0, "Insertion Time"=0, "Cutting Time"=0, "PF Time"=0, "Meas. Time"=0, "Reject Time"=0}, "Measurements"={"1"=0.0, "2"=0.0, "3"=0.0, "4"=0.0}, "Outputs"={"Good Parts"=0, "Reject Parts"=0}, "Cycle Time"=0.0, "Remarks"=""} ("Auto Stats"), Variant=w313) -> (data=w269:T24, error out=w312:errorcluster)
        n117 = Unbundle By Name(w269) -> ("Time-Stamp"=w308:timestamp, "Measurements"=w300:cluster{"1":dbl, "2":dbl, "3":dbl, "4":dbl}, "Outputs"=→"Output Chart":cluster{"Good Parts":u32, "Reject Parts":u32}, "Auto Times"=→"Auto Times":T9)
        "Latest Measure." <- w300
        n118 = call "Stats Unbundle.vi"("State"=Logging_FGV."Log Index", "Auto Stats"=w269) -> ("Cycle Time"=→"Cycle Time" →"Total Time":dbl, "Counters"=w304:cluster{"GoodCount":u32, "RejectCount":u32}, "OEE Cluster"=→"OEE Chart" →"OEE 2":T13, "Avg. Cycle Time"=w282:dbl, "Total Times"=w290:T36, "path"=→"path":path)  [unwired: 3 in, 1 out]
        "Avg. Time" <- w282
        n119 = Format Date/Time String(time format string (%c)="%d-%m-%Y | %H:%M:%S%3u", seconds (now)=w308) -> (date/time string=→"Timestamp":string)  [unwired: 1 in]
        n120 = Unbundle By Name(w280) -> ("Auto Para.Measur. Delays"=w279:dbl[])
        n121 = Unbundle By Name(w304) -> ("GoodCount"=w292:u32, "RejectCount"=w293:u32)
        "Rejects" <- w293
        "Good" <- w292
        "Good Count" <- w292
        "Reject Count" <- w293
        n122 = call "Auto-Pause Check.vi"("Auto Stats"=w269, "Queue"=w270, "Autopause"=w272) -> ("Autopause out"=w271:cluster{"GoodPause":u32, "RejectPause":u32})  [unwired: 8 in]
        n123 = Index Array(array=w279, index #1=1 ("index"), index #2=2 ("index")) -> (element #1=w274:dbl, element #2=w273:dbl)
        n124 = Unbundle(w290) -> ("Index"=w289:dbl, "TF"=w288:dbl, "Insert"=w287:dbl, "Cutting"=w286:dbl, "PF"=w285:dbl, "Measure."=w284:dbl, "Reject"=w283:dbl)
        n125 = Bundle("Index"=w289, "TF"=w288, "Insert"=w287, "Cutting"=w286, "PF"=w285, "Measure."=w284, "Reject"=w283, "Avg. Cycle Time"=w282) -> (→"Time Chart":T12)  [unwired: 1 in]
        n126 = Add(x=w274, y=w273) -> (x+y=w276:dbl)
        n127 = Subtract(x=w274, y=w273) -> (x-y=w275:dbl)
        n128 = Add(x=w292, y=w293) -> (x+y=→"Total Count 2":u32)
        n129 = Unbundle(w300) -> ("1"=w299:dbl, "2"=w298:dbl, "3"=w297:dbl, "4"=w296:dbl)
        n130 = Bundle("1"=w299, "2"=w298, "3"=w297, "4"=w296, w276, w275) -> (→"Measurement Chart":T37)  [unwired: 1 in]
        n131 = Merge Errors(w312) -> (w315:errorcluster)
      }
      frame "Run Manual" {
        # "Update Manual mode"
        n132 = Bundle("Manual Para"="Manual Para", "Reject Pallets"="Reject Pallets") -> (w320:T38)  [unwired: 1 in]
        n133 = for {
          tunnel: w323 -> [w331] mode=indexing
          tunnel: T21."Disabled and Grayed Out" ("Disabled") -> [w330]
          n134 = property class="Bool"(reference=w331, "DisabledEnum"=w330) -> ()  [unwired: 1 in, 2 out]
        }
        n135 = call "Write NS (HMI).vi"("error in (no error)"=w326, "Message Data"=w320, "Message"="Manual Run") -> ("error out"=w325:errorcluster)  [unwired: 8 in]
        n136 = Merge Errors(w325) -> (w328:errorcluster)
      }
      frame "Manual Status" {
        n137 = Variant To Data(error in=w360, type=T25 {"Auto Times"={"Index Time"=0, "TF Time"=0, "Insertion Time"=0, "Cutting Time"=0, "PF Time"=0, "Meas. Time"=0, "Reject Time"=0}, "Results"={"Measurements"={"1"=0.0, "2"=0.0, "3"=0.0, "4"=0.0}, "Reject Pallets"={"Reject 1"=FALSE, "Reject 2"=FALSE, "Reject 3"=FALSE, "Reject 4"=FALSE}}, "OutputCount"=0, "error out"={"status"=FALSE, "code"=0, "source"=""}} ("cluster"), Variant=w359) -> (data=w356:T25, error out=w351:errorcluster)
        n138 = Unbundle(w356) -> ("Auto Times"=w355:T9, "Results"=w347:T39, "OutputCount"=w346:u32, "error out"=w349:errorcluster)
        n139 = for {
          tunnel: w357 -> [w366] mode=indexing
          tunnel: T21."Enabled" ("Disabled") -> [w365]
          n140 = property class="Bool"(reference=w366, "DisabledEnum"=w365) -> ()  [unwired: 1 in, 2 out]
        }
        n141 = Unbundle(w347) -> ("Measurements"=w335:cluster{"1":dbl, "2":dbl, "3":dbl, "4":dbl}, "Reject Pallets"=w336:T3)
        "Measurements" <- w335
        n142 = Bundle("Auto Times"=w355, "error out"=w349) -> (→"Status 2":T10)  [unwired: 1 in]
        n143 = Bundle("Reject Pallets"=w336, "Measurements"=w335) -> (w334:T40)  [unwired: 1 in]
        n144 = call "Counts Update (manual).vi"("output cluster"=w334, "Desired Cycle Time (s)"="Ideal Time", "AVL"="AVL", "OutputCount"=w346, "Counts in"=w350) -> ("OEE"=w340:T13, "Counts out"=w345:cluster{"OutputCount":u32, "RejectCount":u32})  [unwired: 5 in]
        n145 = Unbundle(w340) -> ("PRF"=→"PRF":dbl, "QUA"=→"QUA":dbl, "OEE"=→"OEE":dbl)  [unwired: 1 out]
        n146 = Unbundle(w345) -> ("OutputCount"=→"Output Count":u32, "RejectCount"=→"Rejects 2":u32)
        n147 = case shown="True" "Continuous?" {
          tunnel: w352 -> [_ w364]
          tunnel: w349 -> [_ w363]
          frame False {
          }
          frame True {
            # "Run if continuous is TRUE & No Error"
            n148 = call-poly "Enqueue Message.vi"("error in (no error)"=w363, "Message"="Run Manual", "Message Queue"=w364) -> ()  [unwired: 7 in, 2 out]
          }
        }
      }
      frame "Reset Manual Count" {
        w369 = u32 0 ("Rejects")
        n149 = local write "Rejects 2"(w369) -> ()
        n150 = local write "Output Count"(w369) -> ()
      }
      frame "Reset AutoPause" {
        n151 = Variant To Data(error in=w380, type="" ("Message"), Variant=w378) -> (data=w376:string, error out=w379:errorcluster)
        n152 = case shown="\"ResetRejectCount\", Default" w376 {
          tunnel: w375 -> [w387 w392]
          tunnel: [w386 w391] -> w374
          tunnel: w373 -> [w385 w390]
          frame "ResetGoodCount" {
            n153 = Unbundle By Name(w385) -> ("General Para 2.OutputPause"=w384:dbl)
            n154 = To Unsigned Long Integer(number=w384) -> (unsigned 32bit integer=w383:u32)
            n155 = Bundle By Name(cluster=w387, "GoodPause"=w383) -> (w386:cluster{"GoodPause":u32, "RejectPause":u32})
          }
          frame "ResetRejectCount", Default {
            n156 = Unbundle By Name(w390) -> ("General Para 2.RejectPause"=w389:dbl)
            n157 = To Unsigned Long Integer(number=w389) -> (unsigned 32bit integer=w388:u32)
            n158 = Bundle By Name(cluster=w392, "RejectPause"=w388) -> (w391:cluster{"GoodPause":u32, "RejectPause":u32})
          }
        }
      }
      frame "Error" {
        w398 = 128  # call and forget
        # "Run async so that this loop will continue to run"
        # "Error"
        n159 = Variant To Data(error in=w417, type=errorcluster {"status"=FALSE, "code"=0, "source"=""} ("error constant"), Variant=w415) -> (data=w410:errorcluster, error out=w413:errorcluster)
        n160 = Unbundle By Name(w410) -> ("source"=w409:string)
        n161 = vi-ref "NewDialog.vi"() -> (w405:refnum<vi>)
        n162 = property class="VI"(reference=w405) -> (error out=w407:errorcluster, "Name"=w406:string)  [unwired: 1 in, 1 out]
        n163 = Search and Replace String(input string=w409, search string="<err>") -> (result string=w397:string)  [unwired: 6 in, 3 out]
        n164 = Open VI Reference(type specifier VI Refnum (for type only)=refnum<vi> refnum, vi path=w406, options=w398, error in (no error)=w407) -> (vi reference=w400:refnum<vi>, error out=w401:errorcluster)  [unwired: 2 in]
        n165 = call-by-ref "Start Asynchronous Call"(reference=w400, error in=w401, "inIcon"=T26."Error", "inTitle"="ERROR", "inMessage"=w397) -> (reference out=w403:refnum<vi>, error out=w402:errorcluster)  [unwired: 6 in, 3 out]
        n166 = Close Reference(reference=w403, error in (no error)=w402) -> (error out=w404:errorcluster)
        n167 = call <vilib>:"Simple Error Handler.vi"("error in (no error)"=w404) -> ()  [unwired: 4 in, 5 out]
        n168 = Merge Errors(w413) -> (w412:errorcluster)
      }
      frame "Reject Pause" {
        w423 = 128  # call and forget
        # "Run async so that this loop will continue to run"
        # "Error"
        n169 = Variant To Data(error in=w442, type=errorcluster {"status"=FALSE, "code"=0, "source"=""} ("error constant"), Variant=w440) -> (data=w435:errorcluster, error out=w438:errorcluster)
        n170 = Unbundle By Name(w435) -> ("source"=w434:string)
        n171 = vi-ref "NewDialog.vi"() -> (w430:refnum<vi>)
        n172 = property class="VI"(reference=w430) -> (error out=w432:errorcluster, "Name"=w431:string)  [unwired: 1 in, 1 out]
        n173 = Search and Replace String(input string=w434, search string="<err>") -> (result string=w422:string)  [unwired: 6 in, 3 out]
        n174 = Open VI Reference(type specifier VI Refnum (for type only)=refnum<vi> refnum, vi path=w431, options=w423, error in (no error)=w432) -> (vi reference=w425:refnum<vi>, error out=w426:errorcluster)  [unwired: 2 in]
        n175 = call-by-ref "Start Asynchronous Call"(reference=w425, error in=w426, "inIcon"=T26."Error", "inTitle"="ERROR", "inMessage"=w422) -> (reference out=w428:refnum<vi>, error out=w427:errorcluster)  [unwired: 6 in, 3 out]
        n176 = Close Reference(reference=w428, error in (no error)=w427) -> (error out=w429:errorcluster)
        n177 = call <vilib>:"Simple Error Handler.vi"("error in (no error)"=w429) -> ()  [unwired: 4 in, 5 out]
        n178 = Merge Errors(w438) -> (w437:errorcluster)
      }
      frame "Confirm Quit" {
        # "Confirm Quit - Message that can confirm whether or not the user wants to exit the application."
        n179 = call "NewDialog.vi"("inIcon"=T26."Information", "inTitle"="SHUTDOWN?", "inButton2Text"="Shutdown", "inButton1Text"="", "inMessage"="Are you sure you want to shutdown?") -> ("outButton2"=w445:bool)  [unwired: 4 in, 2 out]
        "Shutdown?" <- w445
        n180 = case shown="True" w445 {
          tunnel: w456 -> [w457 w462]
          tunnel: [w457 w461] -> w453
          tunnel: w452 -> [_ w460]
          frame False {
          }
          frame True {
            n181 = call-poly "Enqueue Message.vi"("Priority Message? (F)"=TRUE, "error in (no error)"=w462, "Message"="Exit", "Message Queue"=w460) -> ("error out"=w461:errorcluster)  [unwired: 6 in, 1 out]
          }
        }
        n182 = Merge Errors(w453) -> (w454:errorcluster)
      }
      frame "Exit" {
        # "Stop the VI"
        # "Release the message queue reference"
        # "Exit - Exit the application."
        n183 = Variant To Data(type=errorcluster {"status"=FALSE, "code"=0, "source"=""} ("error constant"), Variant=w469) -> (data=w470:errorcluster)  [unwired: 1 in, 1 out]
        n184 = call <vilib>:"Simple Error Handler.vi"("error in (no error)"=w470) -> ()  [unwired: 4 in, 5 out]
        n185 = Send Notification(notification=TRUE, notifier=w468) -> (error out=w466:errorcluster)  [unwired: 1 in, 1 out]
        n186 = call "Fire User Event - Stop.vi"("User Event - Stop"=w474) -> ("error out"=w473:errorcluster)  [unwired: 10 in]
        n187 = Release Queue(queue=w479, error in (no error)=w472) -> (error out=w476:errorcluster)  [unwired: 1 in, 2 out]
        n188 = Merge Errors(w466, w473, w476) -> (w475:errorcluster)
      }
      frame Default {
        # "'Default' case only runs if there is a message that isn't defined in any of the other cases.  Output a programming error."
        n189 = xnode "Error Ring"("parameter 0"=w483) -> ("error out"=w484:errorcluster)
      }
    }
    n190 = call "Error Handler - Message Handling Loop.vi"("error in (no error)"=w64, "Message Queue"=w66) -> ("dup error in"=w65:errorcluster)  [unwired: 8 in, 1 out]
  }
  n191 = while {
    tunnel: w34 -> [w501]
    shift-right: [w499] -> w40
    shift-left: w37 -> [w500]
    tunnel: [w495] -> w38
    tunnel: w3 -> [w493]
    stop <- w497 stop-if-true
    # "Event Handling Loop"
    n192 = event shown="[13] \"ResetGoodCount\", \"ResetRejectCount\": Value Change" {
      selector: w500 -> [_ _ _ _ _ _ _ _ _ _ _ _ _ _ _ _ _ _ _ _ _]
      dyn-events: [_ _ _ _ _ _ _ _ _ _ _ _ _ _ _ _ _ _ _ _ _] -> w499
      timeout: 500 -> [_ _ _ _ _ _ _ _ _ _ _ _ _ _ _ _ _ _ _ _ _]
      tunnel: [_ _ _ _ _ _ _ _ _ _ _ _ _ _ _ _ _ _ _ _ TRUE ("Discard?")] -> w497
      tunnel: w501 -> [w506 w510 w522 w527 w531 w535 w539 w543 w548 w553 w562 w586 w590 w594 w599 w601 w604 w635 w644 w653 w655]
      tunnel: [w505 _ _ w526 w530 w534 w538 w542 w547 w552 w561 w587 _ _ w597 w602 w607 _ _ _ _] -> w498
      tunnel: [w504 w510 w522 w525 w529 w533 w537 w541 w546 w551 w560 w586 w590 w594 w598 w601 w603 w635 w644 w653 w655] -> w496
      tunnel: w493 -> [_ _ _ _ _ _ _ _ _ _ w554 _ _ _ _ _ _ _ _ _ _]
      event Panel Close? {
        n193 = event-data() -> ()  [unwired: 1 in, 1 out]
        n194 = call-poly "Enqueue Message.vi"("Priority Message? (F)"=TRUE, "Message"="Exit", "Message Queue"=w506) -> ("error out"=w505:errorcluster, "dup Message Queue"=w504:refnum<queue>)  [unwired: 7 in]
        n195 = event-data("Discard?"=TRUE) -> ()  [unwired: 1 in, 1 out]
      }
      event Timeout {
        n196 = event-data() -> ()  [unwired: 1 in, 1 out]
        n197 = Format Date/Time String(time format string (%c)="%d %b %Y | %I:%M:%S %p") -> (date/time string=→"Date-Time":string)  [unwired: 2 in]
      }
      event "View Log": Value Change {
        w521 = 128  # call and forget
        n198 = event-data() -> ()  [unwired: 1 in, 1 out]
        n199 = local read "path"() -> (w511:path)
        n200 = vi-ref "View Log.vi"() -> (w514:refnum<vi>)
        n201 = property class="VI"(reference=w514) -> (error out=w512:errorcluster, "Name"=w513:string)  [unwired: 1 in, 1 out]
        n202 = Open VI Reference(type specifier VI Refnum (for type only)=refnum<vi> refnum, vi path=w513, options=w521, error in (no error)=w512) -> (vi reference=w519:refnum<vi>, error out=w518:errorcluster)  [unwired: 2 in]
        n203 = call-by-ref "Start Asynchronous Call"(reference=w519, error in=w518, "file path"=w511) -> (reference out=w516:refnum<vi>, error out=w517:errorcluster)  [unwired: 10 in, 1 out]
        n204 = Close Reference(reference=w516, error in (no error)=w517) -> (error out=w515:errorcluster)
        n205 = call <vilib>:"Simple Error Handler.vi"("error in (no error)"=w515) -> ()  [unwired: 4 in, 5 out]
      }
      event "Shutdown": Value Change {
        n206 = event-data() -> ()  [unwired: 1 in, 1 out]
        n207 = call-poly "Enqueue Message.vi"("Priority Message? (F)"=TRUE, "Message"="Confirm Quit", "Message Queue"=w527) -> ("error out"=w526:errorcluster, "dup Message Queue"=w525:refnum<queue>)  [unwired: 7 in]
      }
      event "Home Para", "Home Manual", "Home IOs": Value Change {
        n208 = event-data() -> ()  [unwired: 1 in, 1 out]
        n209 = call-poly "Enqueue Message.vi"("Message"="Initialize", "Message Queue"=w531) -> ("error out"=w530:errorcluster, "dup Message Queue"=w529:refnum<queue>)  [unwired: 8 in]
      }
      event "Back Stats", "Back IO": Value Change {
        n210 = event-data() -> ()  [unwired: 1 in, 1 out]
        n211 = call-poly "Enqueue Message.vi"("Message"="Autocycle Back", "Message Queue"=w535) -> ("error out"=w534:errorcluster, "dup Message Queue"=w533:refnum<queue>)  [unwired: 8 in]
      }
      event "Stats": Value Change {
        n212 = event-data() -> ()  [unwired: 1 in, 1 out]
        n213 = call-poly "Enqueue Message.vi"("Message"="Autocycle Stats", "Message Queue"=w539) -> ("error out"=w538:errorcluster, "dup Message Queue"=w537:refnum<queue>)  [unwired: 8 in]
      }
      event "All IO", "All IOs": Value Change {
        n214 = event-data() -> ()  [unwired: 1 in, 1 out]
        n215 = call-poly "Enqueue Message.vi"("Message"="Autocycle IO", "Message Queue"=w543) -> ("error out"=w542:errorcluster, "dup Message Queue"=w541:refnum<queue>)  [unwired: 8 in]
      }
      event "Home AC": Value Change {
        n216 = event-data() -> ()  [unwired: 1 in, 1 out]
        n217 = call-poly "Enqueue Message.vi"("Message"="Initialize", "Message Queue"=w548) -> ("error out"=w547:errorcluster, "dup Message Queue"=w546:refnum<queue>)  [unwired: 8 in]
        n218 = call "Write NS (HMI).vi"("Message"="Exit Autocycle") -> ()  [unwired: 10 in, 1 out]
      }
      event "Maintenance", "Manual": Value Change {
        n219 = event-data() -> ("CtlRef"=w550:refnum<vi>)  [unwired: 1 in]
        n220 = property class="Bool"(reference=w550) -> ("Label.Text"=w549:string)  [unwired: 1 in, 2 out]
        n221 = call-poly "Enqueue Message.vi"("Message"=w549, "Message Queue"=w553) -> ("error out"=w552:errorcluster, "dup Message Queue"=w551:refnum<queue>)  [unwired: 8 in]
      }
      event "Parameters": Value Change {
        n222 = event-data() -> ("CtlRef"=w559:refnum<vi>)  [unwired: 1 in, 2 out]
        n223 = call "HMI Pop Up Num KP v1.1.vi"("Password Display (F)"=FALSE, "Message In"="Please enter the passcode below:") -> ("Canceled"=w556:bool, "String Out"=w555:string)  [unwired: 8 in]
        n224 = case shown="False" w556 {
          tunnel: w562 -> [w569 w581]
          tunnel: [w568 _] -> w561
          tunnel: [w567 w581] -> w560
          tunnel: w559 -> [w566 _]
          tunnel: w555 -> [w565 _]
          tunnel: w554 -> [w564 _]
          frame False {
            n225 = Equal?(x=w565, y=w564) -> (x = y?=w563:bool)
            n226 = case shown="False" w563 {
              tunnel: w569 -> [w574 w579]
              tunnel: [w573 w578] -> w568
              tunnel: [w572 w577] -> w567
              tunnel: w566 -> [w571 _]
              frame True {
                n227 = property class="Bool"(reference=w571) -> ("Label.Text"=w570:string)  [unwired: 1 in, 2 out]
                n228 = call-poly "Enqueue Message.vi"("Message"=w570, "Message Queue"=w574) -> ("error out"=w573:errorcluster, "dup Message Queue"=w572:refnum<queue>)  [unwired: 8 in]
              }
              frame False {
                n229 = xnode "Error Ring"() -> ("error out"=w575:errorcluster)
                n230 = call-poly "Enqueue Message.vi"("Message Data"=w575, "Message"="Error" ("Message In"), "Message Queue"=w579) -> ("error out"=w578:errorcluster, "dup Message Queue"=w577:refnum<queue>)  [unwired: 7 in]
              }
            }
          }
          frame True {
          }
        }
      }
      event "End Cycle", "Enable Cutting?", "Enable TF?", "Enable PF?", "Enable Index?", "Enable Measure?", "Enable Reject?", "Enable Agitate?", "Enable BF?", "Enable Insertion?": Value Change {
        n231 = event-data() -> ("CtlRef"=w588:refnum<vi>, "NewVal"=w582:bool)  [unwired: 1 in, 1 out]
        n232 = property class="Bool"(reference=w588) -> ("Label.Text"=w585:string)  [unwired: 1 in, 2 out]
        n233 = Concatenate Strings("GV:" ("string"), w585) -> (w583:string)
        n234 = call "Write NS (HMI).vi"("Message Data"=w582, "Message"=w583) -> ("error out"=w587:errorcluster)  [unwired: 9 in]
      }
      event "Reset MCount": Value Change {
        n235 = event-data() -> ()  [unwired: 1 in, 6 out]
        n236 = call-poly "Enqueue Message.vi"("Message"="Reset Manual Count", "Message Queue"=w590) -> ()  [unwired: 8 in, 2 out]
      }
      event "ResetGoodCount", "ResetRejectCount": Value Change {
        n237 = event-data() -> ("CtlRef"=w592:refnum<vi>)  [unwired: 1 in]
        n238 = property class="Bool"(reference=w592) -> ("Label.Text"=w591:string)  [unwired: 1 in, 2 out]
        n239 = call-poly "Enqueue Message.vi"("Message Data"=w591, "Message"="Reset AutoPause", "Message Queue"=w594) -> ()  [unwired: 7 in, 2 out]
      }
      event "Run Manual": Value Change {
        n240 = event-data() -> ("CtlRef"=w596:refnum<vi>)  [unwired: 1 in, 2 out]
        n241 = property class="Bool"(reference=w596) -> ("Label.Text"=w595:string)  [unwired: 1 in, 2 out]
        n242 = call-poly "Enqueue Message.vi"("Message"=w595, "Message Queue"=w599) -> ("error out"=w597:errorcluster, "dup Message Queue"=w598:refnum<queue>)  [unwired: 8 in]
      }
      event "Toggle Motor": Value Change {
        n243 = event-data() -> ()  [unwired: 1 in, 3 out]
        n244 = call "Write NS (HMI).vi"("Message"="Toggle Motor") -> ("error out"=w602:errorcluster)  [unwired: 10 in]
      }
      event "Save Para": Value Change {
        n245 = event-data() -> ()  [unwired: 1 in, 3 out]
        n246 = Cluster To Array(cluster="Agitator Para") -> (array=w624:u32[])
        n247 = Cluster To Array(cluster="Tube Feeder Para") -> (array=w622:u32[])
        n248 = Cluster To Array(cluster="Insertion Para") -> (array=w620:u32[])
        n249 = Cluster To Array(cluster="Cutting Para") -> (array=w618:u32[])
        n250 = Cluster To Array(cluster="PF Para") -> (array=w616:u32[])
        n251 = Cluster To Array(cluster="Meas. Para") -> (array=w614:dbl[])
        n252 = Cluster To Array(cluster="Reject Para") -> (array=w612:u32[])
        n253 = Cluster To Array(cluster="BF Para") -> (array=w610:u32[])
        n254 = Bundle By Name(cluster=T2 {"Agitator Delays"=[1000], "TF Delays"=[1000], "Insertion Delays"=[1000], "Cutting Delays"=[1000], "PF Delays"=[1000], "Measur. Delays"=[1000.0], "Reject Delays"=[1000], "BF Delays"=[1000]} ("Auto Para"), "Agitator Delays"=w624, "TF Delays"=w622, "Insertion Delays"=w620, "Cutting Delays"=w618, "PF Delays"=w616, "Measur. Delays"=w614, "Reject Delays"=w612, "BF Delays"=w610) -> (w609:T2)
        n255 = Bundle("Auto Para"=w609, "General Para"="General Para") -> (w606:cluster{"Auto Para":T2, "General Para":T1})  [unwired: 1 in]
        n256 = property on="Auto Para" class="Clust (strict)"("Value"=w609) -> ()  [unwired: 2 in, 2 out]
        n257 = call-poly "Enqueue Message.vi"("Message Data"=w606, "Message"="Update Para", "Message Queue"=w604) -> ("error out"=w607:errorcluster, "dup Message Queue"=w603:refnum<queue>)  [unwired: 7 in]
      }
      event "Insertion Para.Delay 1", "Insertion Para.Delay 2", "Agitator Para.Delay", "Agitator Para.Timeout", "Cutting Para.Delay", "Cutting Para.Delay 2", "Cutting Para.Delay 3", "Tube Feeder Para.Delay", "Tube Feeder Para.Delay 2", "Tube Feeder Para.Max Attempts", "PF Para.Delay", "PF Para.Timeout", "Reject Para.Delay", "BF Para.Delay 1", "BF Para.Delay 2": Mouse Up {
        n258 = event-data() -> ("CtlRef"=w627:refnum<vi>)  [unwired: 1 in, 4 out]
        n259 = property class="DigNum (strict)"(reference=w627) -> (reference out=w630:refnum<vi>, "Value"=w631:u32)  [unwired: 1 in, 1 out]
        n260 = Number To Fractional String(number=w631, precision (6)=0.0 ("width (-)")) -> (F-format string=w629:string)  [unwired: 2 in]
        n261 = call "HMI Pop Up Num KP v1.1.vi"("String In"=w629) -> ("String Out"=w628:string)  [unwired: 9 in, 1 out]
        n262 = Fract/Exp String To Number(string=w628, default (0 dbl)=0.0 ("default (0 I32)")) -> (number=w633:dbl)  [unwired: 2 in, 1 out]
        n263 = property class="DigNum (strict)"(reference=w630, "Value"=w633) -> ()  [unwired: 1 in, 2 out]
      }
      event "Meas. Para.Delay": Mouse Up {
        n264 = event-data() -> ("CtlRef"=w636:refnum<vi>)  [unwired: 1 in, 4 out]
        n265 = property class="DigNum (strict)"(reference=w636) -> (reference out=w639:refnum<vi>, "Value"=w640:dbl)  [unwired: 1 in, 1 out]
        n266 = Number To Fractional String(number=w640, precision (6)=0.0 ("width (-)")) -> (F-format string=w638:string)  [unwired: 2 in]
        n267 = call "HMI Pop Up Num KP v1.1.vi"("String In"=w638) -> ("String Out"=w637:string)  [unwired: 9 in, 1 out]
        n268 = Fract/Exp String To Number(string=w637, default (0 dbl)=0.0 ("default (0 I32)")) -> (number=w642:dbl)  [unwired: 2 in, 1 out]
        n269 = property class="DigNum (strict)"(reference=w639, "Value"=w642) -> ()  [unwired: 1 in, 2 out]
      }
      event "Meas. Para.Mean Length", "Meas. Para.Tolerance": Mouse Up {
        n270 = event-data() -> ("CtlRef"=w645:refnum<vi>)  [unwired: 1 in, 4 out]
        n271 = property class="DigNum (strict)"(reference=w645) -> (reference out=w648:refnum<vi>, "Value"=w649:dbl)  [unwired: 1 in, 1 out]
        n272 = Number To Fractional String(number=w649, precision (6)=2.0 ("width (-)")) -> (F-format string=w647:string)  [unwired: 2 in]
        n273 = call "HMI Pop Up Num KP v1.1.vi"("String In"=w647) -> ("String Out"=w646:string)  [unwired: 9 in, 1 out]
        n274 = Fract/Exp String To Number(string=w646, default (0 dbl)=0.0 ("default (0 I32)")) -> (number=w651:dbl)  [unwired: 2 in, 1 out]
        n275 = property class="DigNum (strict)"(reference=w648, "Value"=w651) -> ()  [unwired: 1 in, 2 out]
      }
      event User Event {
        # "The Message Handling Loop processed an \"Exit\" message, which fired this event to stop the Event Handling Loop."
        n276 = event-data() -> ()  [unwired: 1 in, 1 out]
      }
    }
    n277 = call "Error Handler - Event Handling Loop.vi"("error in (no error)"=w498, "Message Queue"=w496) -> ("dup error in"=w495:errorcluster)  [unwired: 8 in, 1 out]
  }
  n278 = call "HMI-cRIO Connection Manager.vi"("error in"=w2, "notifier in"=w8, "Queue in"=w34) -> ("error out"=w28:errorcluster, "Notifier out"=w29:refnum<notifier>)  [unwired: 7 in]
  n279 = Unregister For Events(event registration refnum=w40, error in=w38) -> (error out=w41:errorcluster)
  n280 = Merge Errors(w41, w43, w28) -> (w42:errorcluster)
  n281 = call "Destroy User Event - Stop.vi"("error in (no error)"=w42, "User Event - Stop"=w36) -> ("error out"=w31:errorcluster)  [unwired: 9 in]
  n282 = Release Notifier(notifier=w29, error in (no error)=w31) -> (error out=w30:errorcluster)  [unwired: 1 in, 2 out]
  n283 = disable-structure shown="RUN_TIME_ENGINE==True" {
    disable-tunnel: w30 -> [_ _]
    frame condition #0 (active) {
    }
    frame condition #1 {
      n284 = local read "Shutdown?"() -> (w656:bool)
      n285 = case shown="True" w656 {
        tunnel: [_ w658] -> w657
        frame False {
        }
        frame True {
          n286 = call <vilib>:"System Exec.vi"("wait until completion? (T)"=TRUE, "command line"="Shutdown -s -f -t 10") -> ("error out"=w658:errorcluster)  [unwired: 6 in, 3 out]
        }
      }
      n287 = flat-sequence {
        tunnel: w657 -> [_]
        frame #0 {
          n288 = Quit LabVIEW() -> ()  [unwired: 1 in]
        }
      }
    }
  }
